vi "get_status.vi"(0 "VISA resource name in":refnum<visa-resource-name>, 1 "error in":errorcluster) -> (2 "VISA resource name out":refnum<visa-resource-name>, 3 "Status":u8, 4 "error out":errorcluster)   [LabVIEW 2016]
panel:
  # "Status values\n0: Ready Open Loop\n1: Ready Closed Loop\n2: Other"
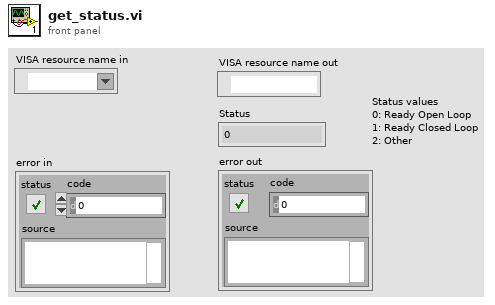
[diagram p1: front panel]
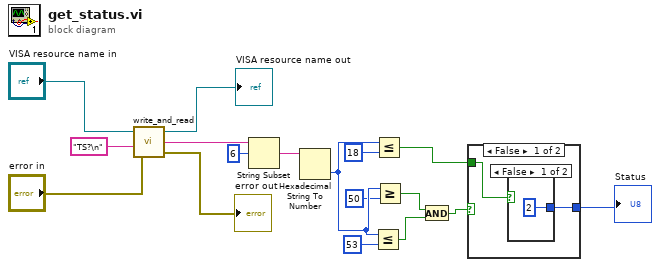
[diagram p0: block diagram]
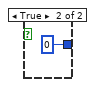
[diagram p2: hidden frame]
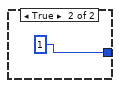
[diagram p3: hidden frame]
diagram:
  n1 = call "write_and_read.vi"("error in"="error in", "write buffer"="TS?\n", "VISA resource name in"="VISA resource name in") -> ("error out"=→"error out":errorcluster, "read buffer"=w12:string, "VISA resource name out"=→"VISA resource name out":refnum<visa-resource-name>)
  n2 = String Subset(string=w12, offset (0)=6) -> (substring=w10:string)  [unwired: 1 in]
  n3 = Hexadecimal String To Number(string=w10) -> (number=w7:u32)  [unwired: 2 in, 1 out]
  n4 = Less Or Equal?(x=w7, y=u32 53) -> (x <= y?=w4:bool)
  n5 = Less Or Equal?(x=w7, y=u32 18) -> (x <= y?=w2:bool)
  n6 = Greater Or Equal?(x=w7, y=u32 50) -> (x >= y?=w5:bool)
  n7 = And(x=w5, y=w4) -> (x .and. y?=w3:bool)
  n8 = case shown="False" w3 {
    tunnel: w2 -> [w19 _]
    tunnel: [w18 1] -> w1
    frame False {
      n9 = case shown="False" w19 {
        tunnel: [2 0] -> w18
        frame False {
        }
        frame True {
        }
      }
    }
    frame True {
    }
  }
  "Status" <- w1
